vi "complex_do_string.vi"(3 "Czy zespolone":bool, 4 "x3":cdb, 5 "x2":cdb, 6 "x1":cdb) -> (0 "x3":string, 1 "x2":string, 2 "x1":string)   [LabVIEW 2020]
doc: "Przekształca liczbę na stringa, oraz pokazuje lub ukrywa część urojoną w zależności od wejścia \"zespolone?\""
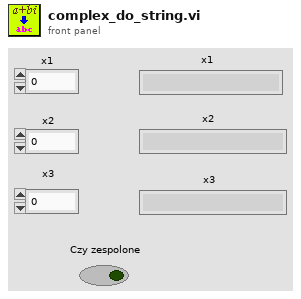
[diagram p1: front panel]
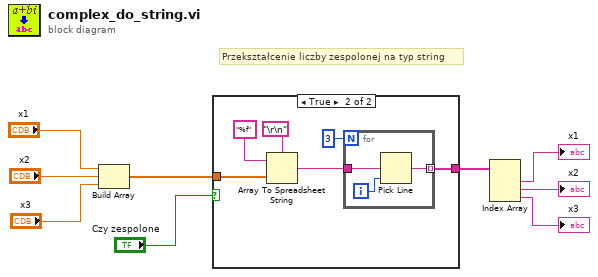
[diagram p0: block diagram]
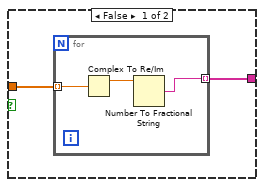
[diagram p2: hidden frame]
diagram:
  # "Przekształcenie liczby zespolonej na typ string"
  n1 = Build Array("x1", "x2", "x3") -> (w6:cdb[])
  n2 = case shown="True" "Czy zespolone" {
    tunnel: w6 -> [w11 w19]
    tunnel: [w10 w15] -> w5
    frame False {
      n3 = for {
        tunnel: w11 -> [w14] mode=indexing
        tunnel: [w12] -> w10 mode=indexing
        n4 = Complex To Re/Im(x + iy=w14) -> (x=w13:dbl)  [unwired: 1 out]
        n5 = Number To Fractional String(number=w13) -> (F-format string=w12:string)  [unwired: 3 in]
      }
    }
    frame True {
      n6 = Array To Spreadsheet String(delimiter (Tab)="\r\n", array=w19, 3:"%f" ("format string")) -> (spreadsheet string=w17:string)
      n7 = for {
        N: 3 -> [_]
        tunnel: w17 -> [w23]
        tunnel: [w22] -> w15 mode=indexing
        i -> [w21]
        n8 = Pick Line(multi-line string=w23, line index=w21) -> (output string=w22:string)  [unwired: 1 in]
      }
    }
  }
  n9 = Index Array(array=w5) -> (element #1=→"x1":string, element #2=→"x2":string, element #3=→"x3":string)  [unwired: 3 in]
